vi "Boot Window.vi"() -> ()   [LabVIEW 2021]
uses:
  <vilib>/Utility/miscctls.llb/LVPointTypeDef.ctl
panel:
  out "Ring":u16(ring)
  # "Loading........"
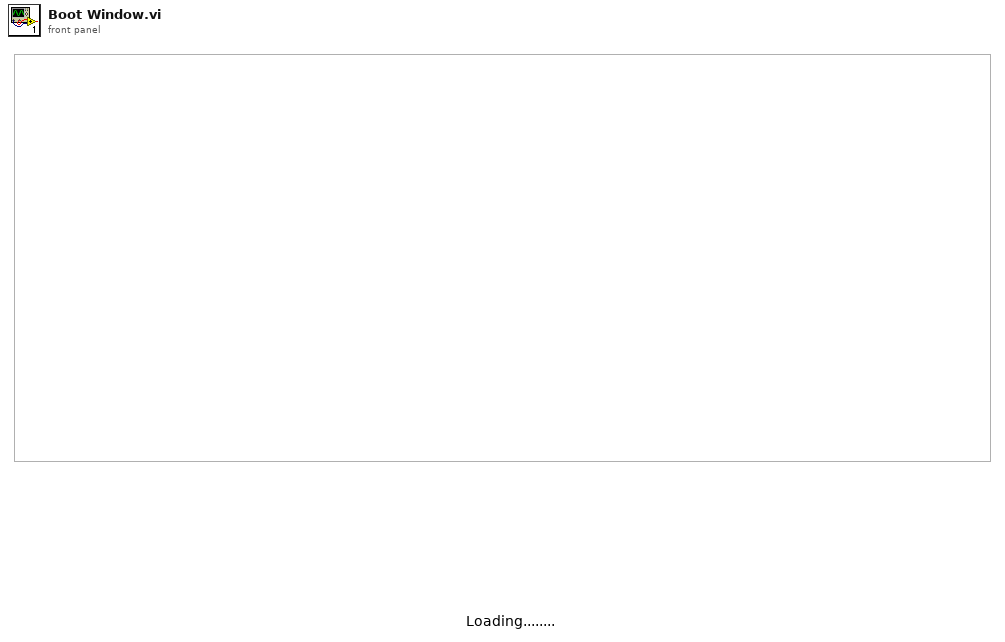
[diagram p1: front panel]
types:
  T1 = typedef "LVPointTypeDef.ctl" = cluster{"Horizontal":i16, "Vertical":i16}
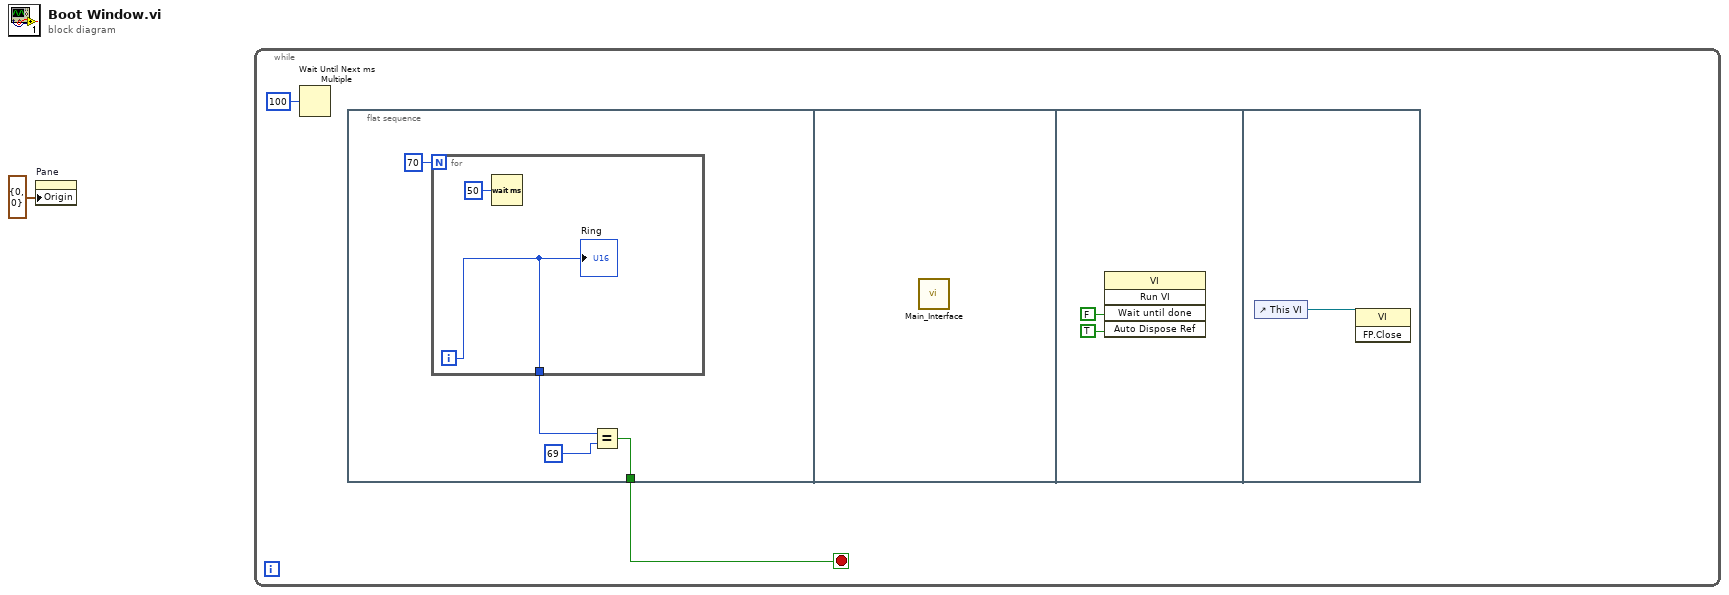
[diagram p0: block diagram]
diagram:
  n1 = property on="Pane" class="Pane"("Origin"=T1 {"Horizontal"=0, "Vertical"=0}) -> ()  [unwired: 2 in, 2 out]
  n2 = while {
    stop <- w3 stop-if-true
    n3 = Wait Until Next ms Multiple(millisecond multiple=u32 100) -> ()  [unwired: 1 out]
    n4 = flat-sequence {
      tunnel: [w4] -> w3
      frame #0 {
        n5 = for {
          N: 70 -> [_]
          tunnel: [w9] -> w6
          i -> [w9]
          n6 = Wait (ms)(milliseconds to wait=u32 50) -> ()  [unwired: 1 out]
          "Ring" <- w9
        }
        n7 = Equal?(x=w6, y=69) -> (x = y?=w4:bool)
      }
      frame #1 {
        n8 = call "Main_Interface.vi"() -> ()  [unwired: 12 in]
      }
      frame #2 {
        n9 = invoke class="VI" method="Run VI"("Wait until done"=FALSE ("Wait Until Done"), "Auto Dispose Ref"=TRUE ("Auto Dispose Reference")) -> ()  [unwired: 3 in, 5 out]
      }
      frame #3 {
        n10 = control-ref of="This VI"() -> (w12:refnum<vi>)
        n11 = invoke class="VI" method="FP.Close"(reference=w12) -> ()  [unwired: 2 in, 3 out]
      }
    }
  }
